vi "Create XLSX.vi"(7 "sheetname":string="Sheet1", 8 "error in (no error)":errorcluster, 10 "File Name":path) -> (0 "error out":errorcluster)   [LabVIEW 2014]
uses:
  C:/Users/LENOVO/Desktop/CodeSpace GUI/LVExcel/Resources/net40/NPOI.OOXML.dll
  Resources/net40/NPOI.OOXML.dll
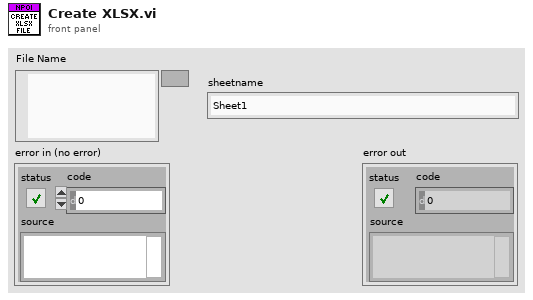
[diagram p1: front panel]
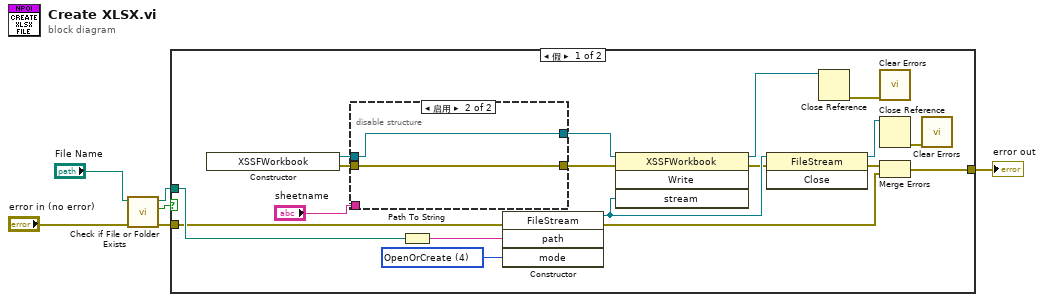
[diagram p0: block diagram]
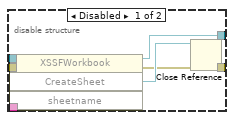
[diagram p2: hidden frame]
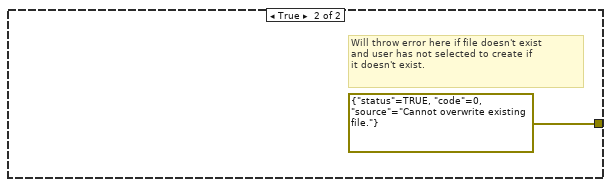
[diagram p3: hidden frame]
diagram:
  n1 = call <vilib>:"Check if File or Folder Exists.vi"("error in (no error)"="error in (no error)", "path"="File Name") -> ("error out"=w2:errorcluster, "file or folder exists?"=w1:bool, "dup path"=w3:path)  [unwired: 7 in]
  n2 = case shown="假" w1 {
    tunnel: [w19 errorcluster {"status"=TRUE, "code"=0, "source"="Cannot overwrite existing file."} ("error IO")] -> w6
    tunnel: w2 -> [w20 _]
    tunnel: w3 -> [w22 _]
    frame False {
      w24 = 4 items=["CreateNew"=1, "Create"=2, "Open"=3, "OpenOrCreate"=4, "Truncate"=5, "Append"=6] ("mode")
      n3 = constructor class="XSSFWorkbook"() -> (reference out=w16:refnum<k24>, error out=w15:errorcluster)  [unwired: 3 in, 1 out]
      n4 = disable-structure shown="启用" {
        disable-tunnel: w16 -> [w29 w33]
        disable-tunnel: w15 -> [w28 w32]
        disable-tunnel: [w27 w33] -> w14
        disable-tunnel: [w26 w32] -> w13
        disable-tunnel: "sheetname" -> [w25 _]
        frame Disabled {
          n5 = invoke class="XSSFWorkbook" method="CreateSheet"(reference=w29, error in=w28, "sheetname"=w25) -> (reference out=w27:refnum<k24>, error out=w30:errorcluster, "CreateSheet"=w31:refnum<k24>)  [unwired: 1 in, 1 out]
          n6 = Close Reference(reference=w31, error in (no error)=w30) -> (error out=w26:errorcluster)
        }
        frame Enabled {
        }
      }
      n7 = Path To String(path=w22) -> (string=w23:string)
      n8 = constructor class="FileStream"(error in=w20, "path"=w23, "mode"=w24) -> (reference out=w11:refnum<k24>, error out=w17:errorcluster)  [unwired: 2 in, 3 out]
      n9 = invoke class="XSSFWorkbook" method="Write"(reference=w14, error in=w13, "stream"=w11) -> (reference out=w21:refnum<k24>, error out=w10:errorcluster)  [unwired: 1 in, 2 out]
      n10 = invoke class="FileStream" method="Close"(reference=w11, error in=w10) -> (reference out=w7:refnum<k24>, error out=w9:errorcluster)  [unwired: 1 in, 1 out]
      n11 = Close Reference(reference=w21) -> (error out=w18:errorcluster)  [unwired: 1 in]
      n12 = call <vilib>:"Clear Errors.vi"("error in (no error)"=w18) -> ()  [unwired: 5 in, 2 out]
      n13 = Close Reference(reference=w7) -> (error out=w8:errorcluster)  [unwired: 1 in]
      n14 = Merge Errors(w9, w17) -> (w19:errorcluster)
      n15 = call <vilib>:"Clear Errors.vi"("error in (no error)"=w8) -> ()  [unwired: 5 in, 2 out]
    }
    frame True {
      # "Will throw error here if file doesn't exist\nand user has not selected to create if\nit doesn't exist."
    }
  }
  "error out" <- w6
